vi "cluster.vi"() -> ()   [LabVIEW 2018]
panel:
  out "output cluster":T1
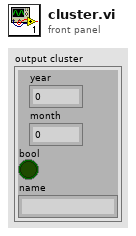
[diagram p1: front panel]
types:
  T1 = cluster{"year":i32, "month":dbl, "bool":bool, "name":string}
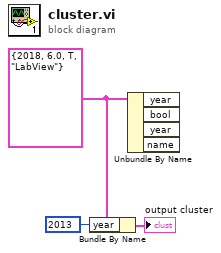
[diagram p0: block diagram]
diagram:
  w3 = T1 {"year"=2018, "month"=6.0, "bool"=TRUE, "name"="LabView"}
  n1 = Bundle By Name(cluster=w3, "year"=2013) -> (→"output cluster":T1)
  n2 = Unbundle By Name(w3) -> ()  [unwired: 4 out]
